vi "Misc_String_ParseROI.vi"(0 "ROI_string":string) -> (4 "ROI":T1)   [LabVIEW 2020]
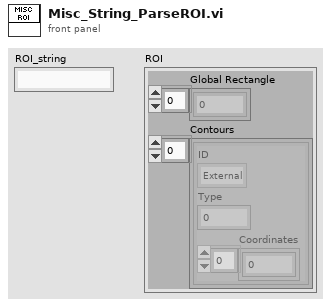
[diagram p1: front panel]
types:
  T1 = cluster{"Global Rectangle":i32[], "Contours":cluster{"ID":enum32{"External", "Internal"}, "Type":u32, "Coordinates":i32[]}[]}
  T2 = cluster{"ID":enum32{"External", "Internal"}, "Type":u32, "Coordinates":i32[]}
  T3 = cluster{"ID":enum32{"External", "Internal"}, "Type":u32, "Coordinates":i32[]}[]
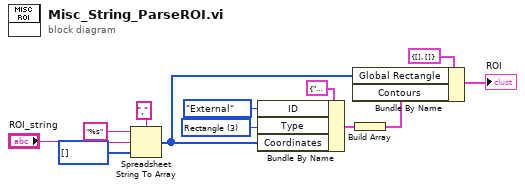
[diagram p0: block diagram]
diagram:
  w8 = u32 3 items=["No Selection", "Point", "Line", "Rectangle", "Oval", "Polygon", "Freehand Region", "Annulus", "Unused2", "Unused3", "Broken Line", "Freehand Line", "Rotated Rectangle"] ("Type")
  n1 = Spreadsheet String To Array(delimiter (Tab)=",", format string="%s", spreadsheet string="ROI_string", array type (2D Dbl)=i32[] [] ("Global Rectangle")) -> (array=w7:i32[])
  n2 = Bundle By Name(cluster=T2 {"ID"=enum."External", "Type"=3, "Coordinates"=[]}, "ID"=enum32{"External", "Internal"}."External", "Type"=w8, "Coordinates"=w7) -> (w6:T2)
  n3 = Build Array(w6) -> (w5:T3)
  n4 = Bundle By Name(cluster=T1 {"Global Rectangle"=[], "Contours"=[]} ("ROI"), "Global Rectangle"=w7, "Contours"=w5) -> (→"ROI":T1)
